vi "play-AFM-CS-imaging_v4_ssx.vi"() -> ()   [LabVIEW 2017]
uses:
  controls/boolean_info.ctl
  controls/TF-params.ctl
  controls/z-axis-params_v4_prescan.ctl
  fpga_VIs/fpga_subVIs_ssxy/fixed-point-ss/typeDefs/FXPControlParams_distEst.ctl
  <vilib>/addons/Control Design/_Model Construction/Model Typedefs.llb/CD State Space Model (MIMO).ctl
  <vilib>/addons/Control Design/_Model Construction/Model Typedefs.llb/CD General Elements.ctl
  <userlib>/_matio/level5/Public/MAT-File Data Types.ctl
  <vilib>/userdefined/High Color/nirio_resource_hc.ctl
  controls/expMetaData_prescan.ctl
  <vilib>/Utility/file.llb/Read Delimited Spreadsheet (DBL).vi
  <vilib>/FPGAPlugInAG/cRIO-9082/niLvFpga_Open_cRIO-9082.vi
  <vilib>/rvi/interface/common/dynamic/niFpgaDynamicAddResources.vi
  <vilib>/FPGAPlugInAG/Dynamic/niLvFpga_Reset_Dynamic.vi
  <vilib>/rvi/interface/common/niFpgaWaitOnOcc.vi
  <vilib>/Utility/error.llb/Error Cluster From Error Code.vi
  <vilib>/rvi/errors/niLvFpgaAdjustHostInterfaceError.vi
  <vilib>/FPGAPlugInAG/Dynamic/niLvFpga_Run_Dynamic.vi
  <vilib>/Utility/file.llb/Write Delimited Spreadsheet (DBL).vi
  <vilib>/FPGAPlugInAG/Dynamic/niLvFpga_Close_Dynamic.vi
  <userlib>/_matio/level5/Public/Write/Append Data Element.llb/Append Data Element (Anything).vi
  <vilib>/rvi/interface/nirviOpenFPGA/nirviOpenFPGA.xnode
  FPGA Bitfiles/afmimagingcontro_FPGATargetSPARTA_cs-scanningv4ssx_nsQOH3rPLfw.lvbitx
  <vilib>/rvi/interface/nirviMethod/nirviMethod.xnode
  <vilib>/rvi/interface/nirviReadWriteControl/nirviReadWriteControl.xnode
  <vilib>/rvi/interface/nirviCloseFPGA/nirviCloseFPGA.xnode
  <vilib>/FPGAPlugInAG/Dynamic/niLvFpga_ConfigureFifo_Dynamic.vi
  <vilib>/rvi/errors/niLvFpgaMergeErrorWithErrorCode.vi
  <vilib>/rvi/interface/Simulation/niFpgaSimulationCallBeginRW.vi
  <vilib>/FPGAPlugInAG/Dynamic/niLvFpga_ReadFifo_Dynamic.vi
  NiFpgaLv.dll
  <userlib>/_matio/level5.lvlib
  <vilib>/FPGAPlugInAG/Dynamic/niLvFpga_WriteFifo_Dynamic.vi
  <vilib>/addons/Control Design/_Model Construction/NI_LinSys_Model Typedefs.lvlib
panel:
  out "num-log-channels":u32
  in  "PID-while-xy-move":bool
  in  "Collect Fan ADC?":bool=TRUE
  out "FAN ADC":dbl[](graph)
  out "ControlMatrices":T1
  out "z-u(k)":sgl
  in  "do-Dz":bool
  in  "TF-params":T2={"TF-order"=2, "Num"=[1.0224493, -2.0410483, 1.0215057, 0.0, 0.0, 0.0, 0.0, 0.0, 0.0], "Den"=[1.0, -1.9962534, 0.9991602, 0.0, 0.0, 0.0, 0.0, 0.0, 0.0]} {"Den" format="%#_12g"; "Num" format="%#_12g"}
  out "boolean \nindicators":T3
  out "CS Time":dbl
  out "Current Case":i16
  out "state times":dbl[](array[numeric])
  out "entity-index":i16
  in  "Tab Control":T4(tab)
  in  "input-data-path":path=path "Z:/afm-cs/imaging/cs-imaging/5microns/parents/cs-traj-512pix-9perc-500nm-5mic-01Hz_250prescan.csv"
  in  "z_axis_params":T5={"TOL"=0.010000002, "z_u_max"=5.0, "setpoint-scan"=-0.3000030517578125, "Ki-scan"=0.02, "uz_safe"=0.0, "Kiz_down"=0.02, "prescan-samples"=250, "setpoint-up"=-0.899993896484375} {"uz_safe" format="%#_13g"; "TOL" format="%#_13g"}
  in  "trigger-0":bool
  in  "numEntities":i16
  out "output-data-path":path
  out "output-meta-data-path":path
  in  "note-blob":string
  in  "overwrite":bool
  in  "TsTicks":u32=1600
  in  "Ki-xy":sgl=0.01
  in  "collect all":bool=TRUE
  in  "zup-err-threshold":fxp<+,24,5>=0.10000228881835938
  in  "xy settled-samples\n threshold":i16=15
  in  "xy error-threshold":sgl=0.01
  in  "control_data_path":path=path "Z:/afm-cs/step-exps/LinControls01.json"
  in  "umax-xy":dbl=3.0 format="%#_13g"
  out "Gdrift-inv-xdir":T6 {"Transport Delay" format="%.2f"; "D" format="%#.5g"; "C" format="%#.5g"; "B" format="%#.5g"; "A" format="%#.5g"; "properties"."Sampling Time" format="%#.6p"; "properties"."Output Delays" format="%.4f"; "properties"."Input Delays" format="%.4f"}
  out "ControlParamsLin-ss":T8={"umax"=3.0, "Ns_obs/cntrl"=0, "ref_f_VEC"=[0.0, 0.0], "du_max"=0.0, "Nbar"=0.0, "Nhyst"=0, "Nsat"=0, "Ndrift+1"=0}
  out "number-settled-samples-x":i16
  out "number-settled-samples-y":i16
  out "case-selected":i16
  out "number-settled-samples-Z":i16
  out "size(s)":i32
  out "y iter":i32
  out "size(s) 2":i32[](array[numeric])
  out "Array":i32[][](array[numeric])
  out "error out 2":errorcluster
  out "z-control":dbl[](graph)
  out "x-axis":dbl[](graph)
  out "z-error":dbl[](graph)
  out "y-axis":dbl[](graph)
  in  "STOP":bool
  # "- If collect all = fasle and collect move = false,\nwe only collect measurement data.\n- If collect all = false, and collect move = true,\nwe collect measurement and move data.\n- If collect all = true, we collect everything."
  # "move"
  # "lower"
  # "z-settle"
  # "scan"
  # "tip-up"
  # "make this come from input csv!"
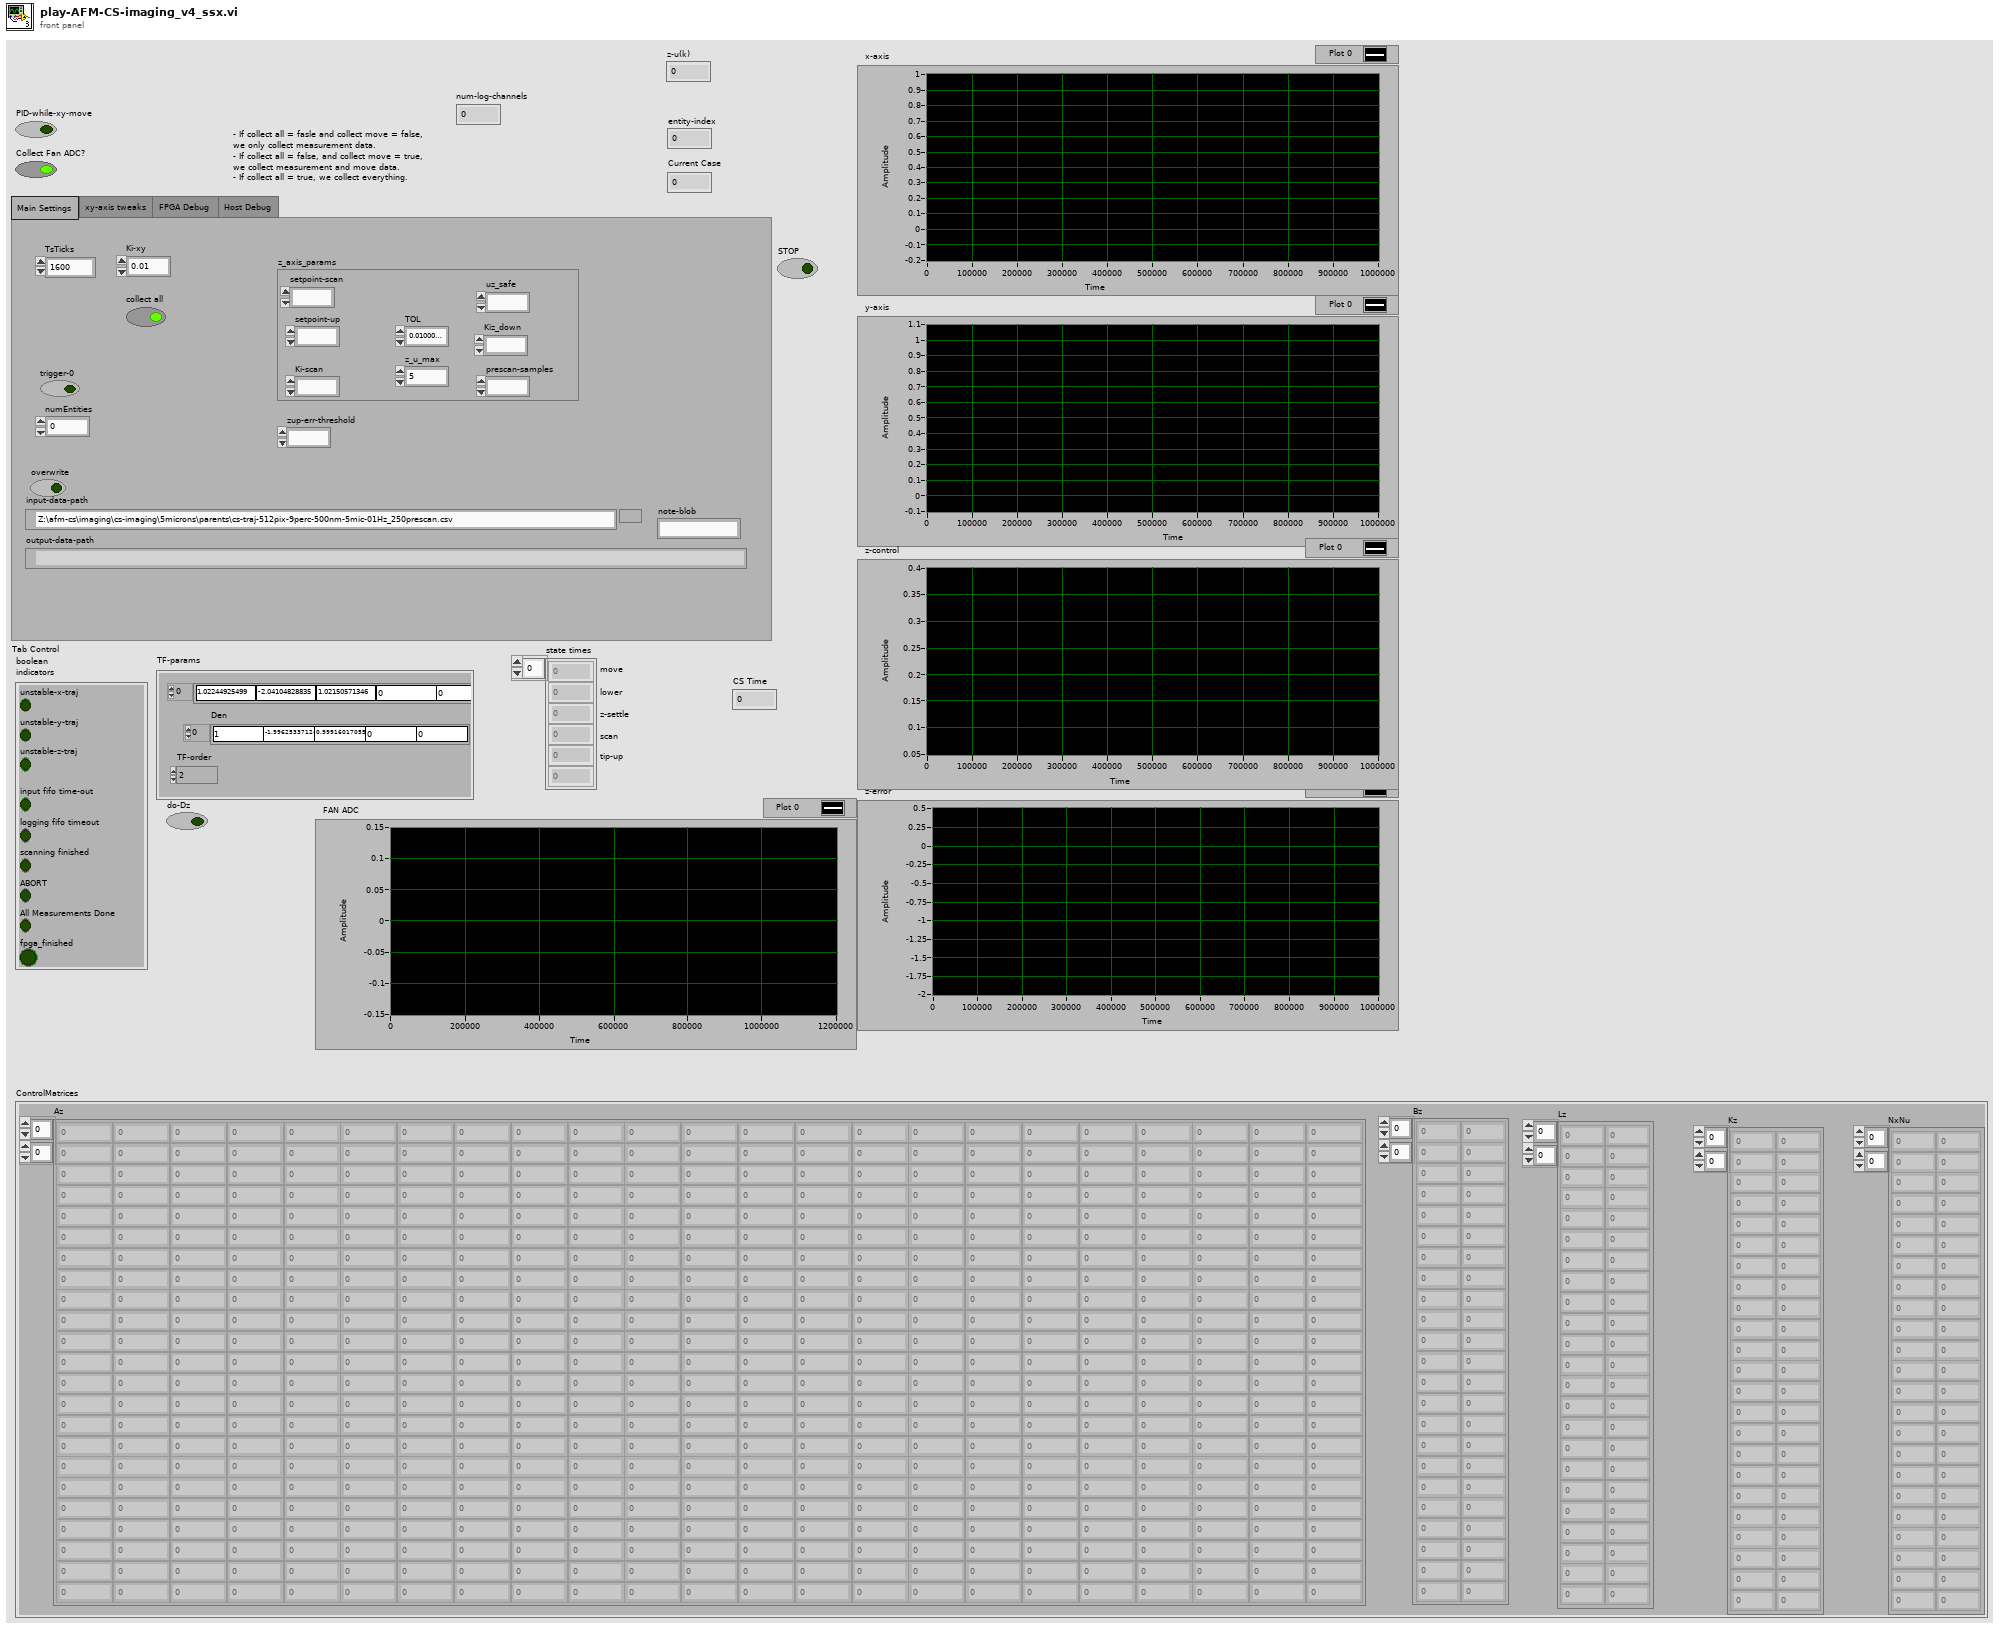
[diagram p1: front panel]
types:
  T1 = cluster{"Az":fxp<+/-,32,4>[][], "Bz":dbl[][], "Lz":dbl[][], "Kz":dbl[][], "NxNu":dbl[][]}
  T2 = typedef "TF-params.ctl" = cluster{"TF-order":i16, "Num":sgl[], "Den":sgl[]}
  T3 = typedef "boolean_info.ctl" = cluster{"unstable-z-traj":bool, "input fifo time-out":bool, "logging fifo timeout":bool, "scanning finished":bool, "unstable-x-traj":bool, "unstable-y-traj":bool, "ABORT":bool, "All Measurements Done":bool, "fpga_finished":bool}
  T4 = enum32{"Main Settings", "xy-axis tweaks", "FPGA Debug ", "Host Debug"}
  T5 = typedef "z-axis-params_v4_prescan.ctl" = cluster{"TOL":sgl, "z_u_max":sgl, "setpoint-scan":fxp<+/-,32,16>, "Ki-scan":sgl, "uz_safe":fxp<+/-,16,5>, "Kiz_down":sgl, "prescan-samples":i16, "setpoint-up":fxp<+/-,32,16>}
  T6 = typedef "NI_LinSys_Model Typedefs.lvlib/CD State Space Model (MIMO).ctl" = cluster{"properties":T7, "A":dbl[][], "B":dbl[][], "C":dbl[][], "D":dbl[][], "StateNames":string[], "Transport Delay":dbl[][]}
  T7 = typedef "NI_LinSys_Model Typedefs.lvlib/CD General Elements.ctl" = cluster{"Model name":string, "Input names":string[], "Output names":string[], "Input Delays":dbl[], "Output Delays":dbl[], "Sampling Time":dbl, "Notes":string}
  T8 = typedef "FXPControlParams_distEst.ctl" = cluster{"umax":fxp<+/-,18,5>, "Ns_obs/cntrl":u8, "ref_f_VEC":fxp<+/-,32,5>[], "du_max":fxp<+/-,18,5>, "Nbar":fxp<+/-,32,5>, "Nhyst":u8, "Nsat":u8, "Ndrift+1":u8}
  T9 = typedef "level5.lvlib/MAT-File Data Types.ctl" = enum32{"_invalid", "miINT8", "miUINT8", "miINT16", "miUINT16", "miINT32", "miUINT32", "miSINGLE", "_reserved_1", "miDOUBLE", "_reserved_2", "_reserved_3", "miINT64", "miUINT64", "miMATRIX", "miCOMPRESSED", "miUTF8", "miUTF16", "miUTF32"}
  T10 = typedef "nirio_resource_hc.ctl" = tag
  T11 = typedef "ObserverMatrices.ctl" = cluster{"Az":fxp<+/-,32,4>[][], "Bz":dbl[][], "Lz":dbl[][], "Kz":dbl[][], "NxNu":dbl[][]}
  T12 = cluster{"unstable-z-traj":bool, "input fifo time-out":bool, "logging fifo timeout":bool, "scanning finished":bool, "unstable-x-traj":bool, "unstable-y-traj":bool, "ABORT":bool, "All Measurements Done":bool, "fpga_finished":bool}
  T13 = typedef "expMetaData_prescan.ctl" = cluster{"xy_error_threshold":sgl, "xy_settled_samples_threshold":i16, "Ki_xy":sgl, "state_counts":dbl[], "TOL":sgl, "z_u_max":sgl, "setpoint-up":sgl, "Ki-scan":sgl, "Z_error_threshold":sgl, "zup_N":i16, "Num":sgl[], "Den":sgl[], "prescan-samples":i16, "Kiz_down":sgl, "do_xy_CL":bool, "do_Alt_Ztrigger":bool, "output-data-path":path, "input-data-path":path, "zup-error-threshold":sgl, "setpoint-scan":sgl, "do_Dz":bool}
  T14 = enum16{"open", "replace", "create", "open or create", "replace or create", "replace or create with confirmation"}
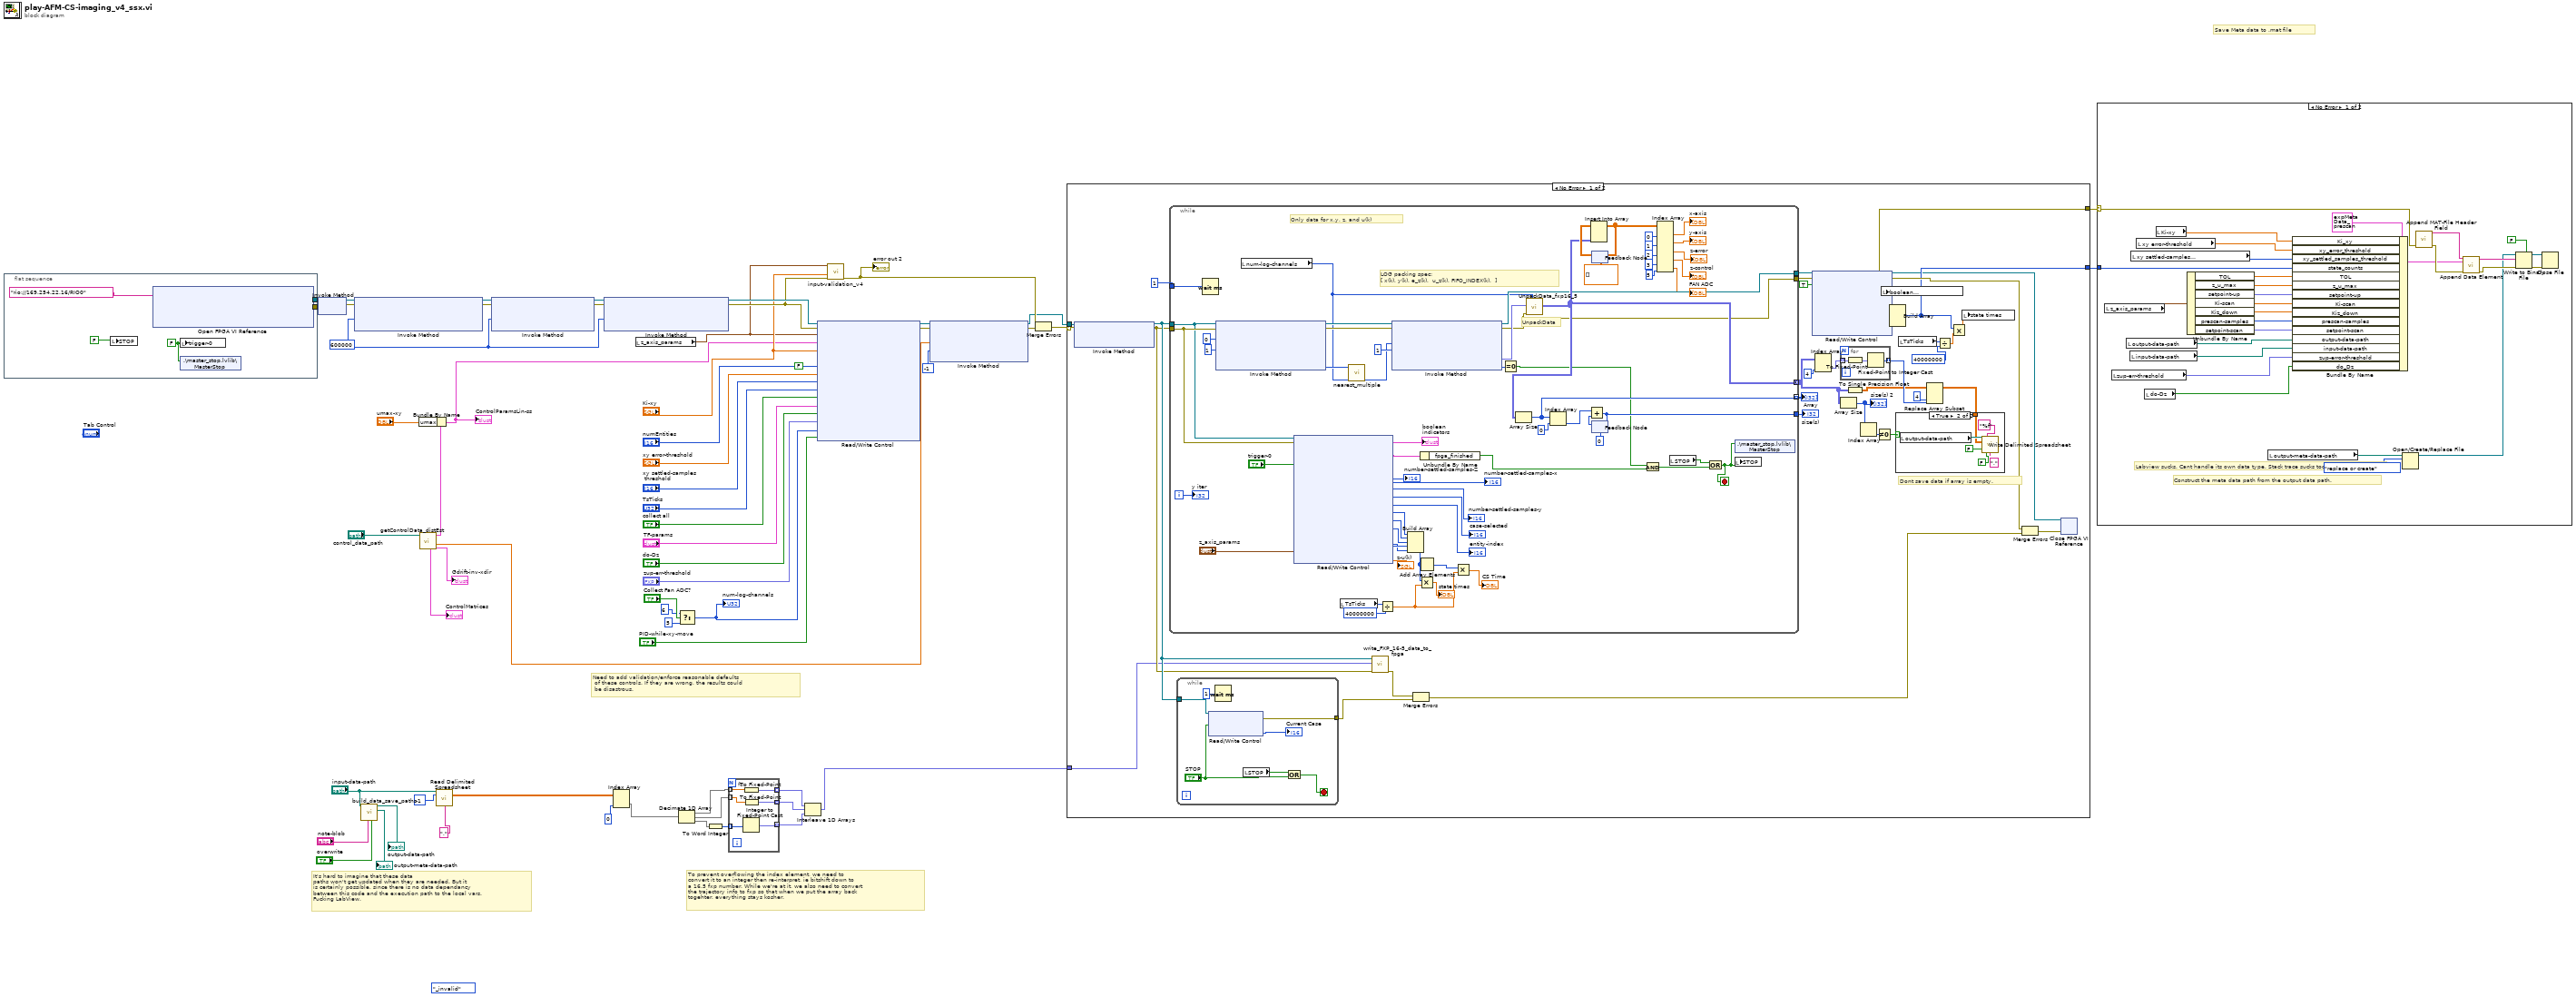
[diagram p0: block diagram]
diagram:
  (unwired) MAT-File_Data_Types."_invalid" ("MAT-File Data Types")
  w19 = 600000
  # "It's hard to imagine that these data\npaths won't get updated when they are needed. But it \nis certainly possible, since there is no data dependancy \nbetween this code and the execution path to the local vars.\nFucking LabView."
  # "Save Meta data to .mat file"
  # "To prevent overflowing the index element, we need to \nconvert it to an integer then re-interpret, ie bitshift down to \na 16,5 fxp number. While we're at it, we also need to convert\nthe trajectory info to fxp so that when we put the array back\ntogehter, everything stays kosher."
  # "Need to add validation/enforce reasonable defaults\n of these controls. If they are wrong, the results could\n be disastrous."
  n1 = flat-sequence {
    tunnel: [w66] -> w60
    tunnel: [w65] -> w59
    frame #0 {
      w62 = FALSE ("trigger-0")
      n2 = local write "STOP"(FALSE) -> ()
      n3 = xnode "Open FPGA VI Reference"("resource name"=T10 "rio://169.254.22.16/RIO0") -> ("FPGA VI Reference Out"=w66:refnum<k20>, "error out"=w65:errorcluster)  [unwired: 1 in]
      n4 = local write "trigger-0"(w62) -> ()
      n5 = shared-variable ".\\master_stop.lvlib\\MasterStop"(w62) -> ()  [unwired: 1 in, 1 out]
    }
  }
  n6 = xnode "Invoke Method"("FPGA VI Reference In"=w60, "error in"=w59) -> ("FPGA VI Reference Out"=w57:refnum<k20>, "error out"=w56:errorcluster)
  n7 = xnode "Invoke Method"("FPGA VI Reference In"=w57, "error in"=w56, "Requested Depth"=w19) -> ("FPGA VI Reference Out"=w20:refnum<k20>, "error out"=w21:errorcluster)  [unwired: 1 out]
  n8 = call "build_data_save_paths.vi"("overwrite"="overwrite", "note-blob"="note-blob", "input-file"="input-data-path") -> ("output-meta-data-path"=→"output-meta-data-path":path, "output-data-path"=→"output-data-path":path)  [unwired: 5 in, 2 out]
  n9 = call "getControlData_distEst.vi"("system data path"="control_data_path") -> ("Gdrift"=→"Gdrift-inv-xdir":T6, "AllMatrix"=w13:dbl[], "ControlParams"=w10:T8, "ControlMatrices"=→"ControlMatrices":T11)  [unwired: 7 in]
  n10 = Bundle By Name(cluster=w10, "umax"="umax-xy") -> (w9:T8)
  "ControlParamsLin-ss" <- w9
  n11 = call-poly <vilib>:"Read Delimited Spreadsheet.vi"("file path (dialog if empty)"="input-data-path", "number of rows (all:-1)"=-1, "delimiter (\\t)"=",") -> ("all rows"=w53:dbl[][])  [unwired: 7 in, 5 out]
  n12 = xnode "Invoke Method"("FPGA VI Reference In"=w20, "error in"=w21, "Requested Depth"=w19) -> ("FPGA VI Reference Out"=w23:refnum<k20>, "error out"=w22:errorcluster)  [unwired: 1 out]
  n13 = xnode "Invoke Method"("FPGA VI Reference In"=w23, "error in"=w22, "Requested Depth"=w19) -> ("FPGA VI Reference Out"=w61:refnum<k20>, "error out"=w27:errorcluster)  [unwired: 1 out]
  n14 = Index Array(array=w53, index (col)=0 ("dimension size")) -> (element=w40:dbl[])  [unwired: 1 in]
  n15 = local read "z_axis_params"() -> (w25:T5)
  n16 = Decimate 1D Array(w40) -> (w46:dbl[], w45:dbl[], w47:dbl[])
  n17 = Select(t=u32 6 ("y"), s="Collect Fan ADC?", f=u32 5 ("y")) -> (s? t:f=w2:u32)
  "num-log-channels" <- w2
  n18 = To Word Integer(number=w47) -> (16bit integer=w44:i16[])
  n19 = for {
    tunnel: w46 -> [w72] mode=indexing
    tunnel: w45 -> [w71] mode=indexing
    tunnel: [w70] -> w42 mode=indexing
    tunnel: [w69] -> w43 mode=indexing
    tunnel: w44 -> [w68] mode=indexing
    tunnel: [w67] -> w41 mode=indexing
    n20 = Integer to Fixed-Point Cast(integer=w68) -> (fixed-point=w67:fxp<+/-,16,5>)  [unwired: 1 in]
    n21 = To Fixed-Point(number=w72) -> (fixed-point=w69:fxp<+/-,16,5>)  [unwired: 1 in]
    n22 = To Fixed-Point(number=w71) -> (fixed-point=w70:fxp<+/-,16,5>)  [unwired: 1 in]
  }
  n23 = Interleave 1D Arrays(w43, w42, w41) -> (w39:fxp<+/-,16,5>[])
  n24 = xnode "Read/Write Control"("FPGA VI Reference In"=w61, "error in"=w27, "z_axis_params"=w25, "ControlParamsLin"=w9, "Ki-xy"="Ki-xy", "trigger-0"=FALSE, "numEntities"="numEntities", "xy-error-threshold"="xy error-threshold", "settled-samples threshold"="xy settled-samples\n threshold", "TsTicks"="TsTicks", "collect all"="collect all", "TF-params"="TF-params", "do-Dz"="do-Dz", "zup-err-threshold"="zup-err-threshold", "num-log-channels"=w2, "PID-while-xy-move"="PID-while-xy-move") -> ("FPGA VI Reference Out"=w17:refnum<k20>, "error out"=w16:errorcluster)
  n25 = call "input-validation_v4.vi"("error constant"=w27, "Ki-xy"="Ki-xy", "z_axis_params"=w25) -> ("error out"=w28:errorcluster)  [unwired: 8 in]
  "error out 2" <- w28
  n26 = xnode "Invoke Method"("FPGA VI Reference In"=w17, "error in"=w16, "Data"=w13, "Timeout (ms)"=-1) -> ("FPGA VI Reference Out"=w14:refnum<k20>, "error out"=w15:errorcluster)  [unwired: 1 out]
  n27 = Merge Errors(w28, w15) -> (w31:errorcluster)
  n28 = case shown="No Error" w31 {
    selector: w31 -> [w79 w189]
    tunnel: w14 -> [w110 _]
    tunnel: w39 -> [w76 _]
    tunnel: [w109 w189] -> w37
    tunnel: [w108 _] -> w36
    frame No Error {
      # "Dont save data if array is empty."
      n29 = xnode "Invoke Method"("FPGA VI Reference In"=w110, "error in"=w79) -> ("FPGA VI Reference Out"=w78:refnum<k20>, "error out"=w77:errorcluster)  [unwired: 1 in]
      n30 = while {
        tunnel: 1 -> [w188]
        tunnel: w78 -> [w177]
        tunnel: w77 -> [w178]
        tunnel: [w150] -> w104
        tunnel: [w156] -> w95 mode=concatenating
        tunnel: [w175] -> w106
        tunnel: [w154] -> w103
        tunnel: [w170] -> w100 mode=indexing
        i -> [w176]
        stop <- w139 stop-if-true
        # "LOG packing spec:\n[ x(k), y(k), e_z(k),  u_z(k), FIFO_INDEX(k),  ]"
        # "Only data for x,y, z, and u(k)"
        # "UnpackData"
        n31 = Wait (ms)(milliseconds to wait=w188) -> ()  [unwired: 1 out]
        n32 = xnode "Invoke Method"("FPGA VI Reference In"=w177, "error in"=w178, "Number of Elements"=0 ("Timeout (ms)"), "Timeout (ms)"=1) -> ("FPGA VI Reference Out"=w184:refnum<k20>, "error out"=w185:errorcluster, "Elements Remaining"=w173:u32)  [unwired: 1 out]
        n33 = local read "num-log-channels"() -> (w128:u32)
        n34 = xnode "Read/Write Control"("FPGA VI Reference In"=w177, "error in"=w178, "trigger-0"="trigger-0", "z_axis_params"="z_axis_params") -> ("boolean  indicators"=w143:T12, "number-settled-samples-Z"=→"number-settled-samples-Z":i16, "number-settled-samples-x"=→"number-settled-samples-x":i16, "number-settled-samples-y"=→"number-settled-samples-y":i16, "Current Case"=→"case-selected":u8, "entity-index"=→"entity-index":i16, "state1-count"=w138:u64, "state2-count"=w137:u64, "state3-count"=w136:u64, "state4-count"=w152:u64, "state5-count"=w151:u64, "z-u(k)"=→"z-u(k)":sgl)  [unwired: 1 in, 2 out]
        "boolean \nindicators" <- w143
        n35 = local read "TsTicks"() -> (w146:u32)
        n36 = call "nearest_multiple.vi"("numChan"=w128, "N"=w173) -> ("(int) y*floor(x/y)"=w172:u64)  [unwired: 9 in]
        n37 = Divide(x=w146, y=u32 40000000) -> (x/y=w141:dbl)
        n38 = xnode "Invoke Method"("FPGA VI Reference In"=w184, "error in"=w185, "Number of Elements"=w172, "Timeout (ms)"=1) -> ("FPGA VI Reference Out"=w150:refnum<k20>, "error out"=w154:errorcluster, "Data"=w155:fxp<+/-,16,5>[], "Elements Remaining"=w134:u32)
        n39 = Build Array(w138, w137, w136, w152, w151) -> (w142:u64[])
        n40 = Add Array Elements(numeric array=w142) -> (sum=w147:u64)
        n41 = Multiply(x=w142, y=w141) -> (x*y=→"state times":dbl[])
        n42 = Unbundle By Name(w143) -> ("fpga_finished"=w133:bool)
        n43 = Multiply(x=w147, y=w141) -> (x*y=→"CS Time":dbl)
        n44 = Equal To 0?(x=w134) -> (x = 0?=w131:bool)
        n45 = call "UnpackData_fxp16_5.vi"("NumChannels"=w128, "error In"=w154, "1D Data In"=w155) -> ("2D Data Out"=w156:fxp<+/-,16,5>[][])  [unwired: 7 in, 1 out]
        n46 = Array Size(array=w156) -> (size(s)=w170:i32[])
        n47 = Index Array(array=w170, index=0) -> (element=w180:i32)
        n48 = feedback #1(0) -> (w181:i32)
        n49 = Add(x=w180, y=w181) -> (x+y=w175:i32)
        n50 = feedback-in #1(w175) -> ()
        n51 = feedback #2(dbl[][] []) -> (w166:dbl[][])
        n52 = Insert Into Array(array=w166, new element=w156) -> (w157:dbl[][])  [unwired: 2 in]
        n53 = feedback-in #2(w157) -> ()
        n54 = And(x=w131, y=w133) -> (x .and. y?=w132:bool)
        n55 = Index Array(array=w157, index (col) #1=0 ("disabled index (col)"), index (col) #2=1 ("index (col)"), index (col) #3=2 ("index (col)"), index (col) #4=3 ("index (col)"), index (col) #5=5 ("index (col)")) -> (element #1=→"x-axis":dbl[], element #2=→"y-axis":dbl[], element #3=→"z-error":dbl[], element #4=→"z-control":dbl[], element #5=→"FAN ADC":dbl[])  [unwired: 5 in]
        n56 = local read "STOP"() -> (w171:bool)
        n57 = Or(x=w171, y=w132) -> (x .or. y?=w139:bool)
        n58 = shared-variable ".\\master_stop.lvlib\\MasterStop"(w139) -> ()  [unwired: 1 in, 1 out]
        n59 = local write "STOP"(w139) -> ()
        "y iter" <- w176
      }
      "size(s)" <- w106
      "Array" <- w100
      n60 = while {
        tunnel: w78 -> [w126]
        tunnel: [w120] -> w75
        stop <- w122 stop-if-true
        n61 = xnode "Read/Write Control"("FPGA VI Reference In"=w126, "ABORT"="STOP") -> ("error out"=w120:errorcluster, "Current Case"=→"Current Case":u8)  [unwired: 1 in, 1 out]
        n62 = Wait (ms)(milliseconds to wait=u32 1) -> ()  [unwired: 1 out]
        n63 = local read "STOP"() -> (w123:bool)
        n64 = Or(x=w123, y="STOP") -> (x .or. y?=w122:bool)
      }
      n65 = call "write_FXP_16-5_data_to_fpga.vi"("error in"=w77, "all rows"=w76, "FPGA Interface"=w78) -> ("error out"=w74:errorcluster)  [unwired: 7 in, 1 out]
      n66 = Merge Errors(w74, w75) -> (w73:errorcluster)
      n67 = xnode "Read/Write Control"("FPGA VI Reference In"=w104, "error in"=w103, "ABORT"=TRUE) -> ("FPGA VI Reference Out"=w101:refnum<k20>, "error out"=w109:errorcluster, "boolean  indicators"=w84:T12, "state1-count"=w93:u64, "state2-count"=w92:u64, "state3-count"=w91:u64, "state4-count"=w90:u64, "state5-count"=w89:u64)
      n68 = Index Array(array=w95, index (col)=4) -> (element=w98:fxp<+/-,16,5>[])  [unwired: 1 in]
      n69 = for {
        tunnel: w98 -> [w118] mode=indexing
        tunnel: [w119] -> w96 mode=indexing
        n70 = To Fixed-Point(number=w118) -> (fixed-point=w117:fxp<+/-,16,5>)  [unwired: 1 in]
        n71 = Fixed-Point to Integer Cast(1:w117) -> (0:w119:i16)
      }
      n72 = Array Size(array=w95) -> (size(s)=w85:i32[])
      "size(s) 2" <- w85
      n73 = To Single Precision Float(number=w95) -> (single precision float=w94:sgl[][])
      n74 = Index Array(array=w85) -> (element=w86:i32)  [unwired: 1 in]
      n75 = Not Equal To 0?(x=w86) -> (x != 0?=w87:bool)
      n76 = local write "boolean \nindicators"(w84) -> ()
      n77 = Build Array(w93, w92, w91, w90, w89) -> (w108:u64[])
      n78 = local read "TsTicks"() -> (w83:u32)
      n79 = Replace Array Subset(array=w94, new element=w96, index (col)=4) -> (w88:sgl[][])  [unwired: 1 in]
      n80 = case shown="True" w87 {
        tunnel: w88 -> [_ w111]
        frame False {
        }
        frame True {
          n81 = local read "output-data-path"() -> (w116:path)
          n82 = call-poly <vilib>:"Write Delimited Spreadsheet.vi"("file path (dialog if empty)"=w116, "format (%.3f)"="%f", "2D data"=w111, "append to file? (new file:F)"=FALSE, "transpose? (no:F)"=FALSE, "delimiter (\\t)"=",") -> ()  [unwired: 8 in, 2 out]
        }
      }
      n83 = Divide(x=w83, y=u32 40000000) -> (x/y=w81:dbl)
      n84 = Multiply(x=w108, y=w81) -> (x*y=w80:dbl[])
      n85 = local write "state times"(w80) -> ()
      n86 = Merge Errors(w109, w73) -> (w105:errorcluster)
      n87 = xnode "Close FPGA VI Reference"("FPGA VI Reference In"=w101, "error in"=w105) -> ()  [unwired: 1 out]
    }
    frame Error {
    }
  }
  n88 = case shown="No Error" w37 {
    selector: w37 -> [w211 _]
    tunnel: w36 -> [w205 _]
    frame No Error {
      # "Construct the meta data path from the output data path."
      # "Labview sucks. Cant handle its own data type. Stack trace sucks too."
      n89 = local read "z_axis_params"() -> (w204:T5)
      n90 = local read "zup-err-threshold"() -> (w191:fxp<+,24,5>)
      n91 = local read "output-data-path"() -> (w197:path)
      n92 = local read "input-data-path"() -> (w198:path)
      n93 = local read "xy settled-samples\n threshold"() -> (w201:i16)
      n94 = local read "xy error-threshold"() -> (w202:sgl)
      n95 = local read "do-Dz"() -> (w190:bool)
      n96 = local read "Ki-xy"() -> (w203:sgl)
      n97 = Unbundle By Name(w204) -> ("TOL"=w208:sgl, "z_u_max"=w207:sgl, "setpoint-up"=w195:fxp<+/-,32,16>, "Ki-scan"=w206:sgl, "Kiz_down"=w194:sgl, "prescan-samples"=w192:i16, "setpoint-scan"=w193:fxp<+/-,32,16>)
      n98 = local read "output-meta-data-path"() -> (w199:path)
      n99 = Bundle By Name(cluster=T13 {"xy_error_threshold"=0.1, "xy_settled_samples_threshold"=200, "Ki_xy"=0.005, "state_counts"=[], "TOL"=0.3, "z_u_max"=5.0, "setpoint-up"=-5e-06, "Ki-scan"=0.001, "Z_error_threshold"=0.0, "zup_N"=5000, "Num"=[-0.00254, 0.000408, 0.00295, 0.0, 0.0, 0.0, 0.0, 0.0, 0.0], "Den"=[0.982758, -1.98194, 1.0, 0.0, 0.0, 0.0, 0.0, 0.0, 0.0], "prescan-samples"=0, "Kiz_down"=0.001, "do_xy_CL"=FALSE, "do_Alt_Ztrigger"=FALSE, "output-data-path"=path "", "input-data-path"=path "", "zup-error-threshold"=0.0, "setpoint-scan"=0.0, "do_Dz"=FALSE} ("ExpMetaData"), "Ki_xy"=w203, "xy_error_threshold"=w202, "xy_settled_samples_threshold"=w201, "state_counts"=w205, "TOL"=w208, "z_u_max"=w207, "setpoint-up"=w195, "Ki-scan"=w206, "Kiz_down"=w194, "prescan-samples"=w192, "setpoint-scan"=w193, "output-data-path"=w197, "input-data-path"=w198, "zup-error-threshold"=w191, "do_Dz"=w190) -> (w209:T13)
      n100 = Open/Create/Replace File(file path (use dialog)=w199, operation (0:open)=T14."replace or create") -> (refnum out=w210:refnum<file>)  [unwired: 4 in, 2 out]
      n101 = call <userlib>:"Append MAT-File Header Field.vi"("error"=w211) -> ("result string"=w218:string, "error out"=w212:errorcluster)  [unwired: 13 in]
      n102 = call-poly <userlib>:"Append Data Element.vi"("initial string"=w218, "data"=w209, "error in (no error)"=w212) -> ("result string"=w216:string, "error out"=w217:errorcluster)  [unwired: 11 in]
      n103 = Write to Binary File(file (use dialog)=w210, data=w216, error in=w217, 5:FALSE ("prepend array or string size? (T)")) -> (refnum out=w213:refnum<file>, error out=w214:errorcluster)  [unwired: 2 in, 1 out]
      n104 = Close File(refnum=w213, error in=w214) -> ()  [unwired: 2 out]
    }
    frame Error {
    }
  }
